vi "Phase III monitor screen.vi"() -> ()   [LabVIEW 2022 SP3]
panel:
  out "C bottom open circuit - LOX":bool
  out "C top open circuit -LOX":bool
  out "B top open circuit - LOX":bool
  out "B Top Open circuit - LOX":bool
  out "A bottom open circuit -LOX":bool
  out "A Top Open circuit -LOX":bool
  out "C Bottom  Short Circuit - ATF 2":bool
  out "C top Short Circuit - LOX":bool
  out "B Bottom short circuit - LOX":bool
  out "B top Short circuit - LOX":bool
  out "A bottom short circuit - LOX":bool
  out "A top Short Circuit - LOX":bool
  out "Speed cmd & Response mismatch- LOX":bool
  out "Motor overload - LOX":bool
  out "Over temperature - LOX":bool
  out "Over speed - LOX":bool
  out "C Phase Short circuit - LOX":bool
  out "C Phase open circuit -LOX":bool
  out "B Phase Short circuit - LOX":bool
  out "B Phase open circuit-LOX":bool
  out "A phase short circuit-LOX":bool
  out "A Phase open circuit -LOX":bool
  in  "Ia,ph,Mean  5":dbl format="%#_g A"
  in  "Ia,ph,Mean  4":dbl format="%#_g A"
  in  "DC Busbar 5":dbl format="%#_g K"
  in  "Ia,ph,Mean  2":dbl format="%#_g A"
  in  "Ic,ph,rms":dbl format="%#_g A"
  in  "Ib,ph,rms":dbl format="%#_g A"
  in  "Ia,ph,rms":dbl format="%#_g A"
  in  "Idc":dbl format="%#_g A"
  in  "Vc,ph,Mean 2":dbl format="%#_g V"
  in  "Vb,ph,Mean 2":dbl format="%#_g V"
  in  "Va,ph,Mean 2":dbl format="%#_g V"
  in  "Vc,ph,rms":dbl format="%#_g V"
  in  "Vb,ph,rms 2":dbl format="%#_g V"
  in  "Va,ph,rms 2":dbl format="%#_g V"
  in  "Vdc":dbl format="%#_g V"
  in  "DC Busbar 4":dbl format="%#_g K"
  in  "DC Busbar 3":dbl format="%#_g K"
  in  "Leg3 CJ":dbl format="%#_g K"
  in  "Leg2 CJ":dbl format="%#_g K"
  in  "Leg1 CJ":dbl format="%#_g K"
  in  "Ia,ph,Mean  3":dbl format="%#_g A"
  in  "Ia,ph,Mean  2":dbl format="%#_g A"
  in  "DC Busbar 2":dbl format="%#_g K"
  out "C bottom open circuit - ATF":bool
  out "C top open circuit -ATF":bool
  out "B top open circuit - ATF":bool
  out "B Top Open circuit - ATF":bool
  out "A bottom open circuit -ATF":bool
  out "A Top Open circuit -ATF":bool
  out "C Bottom  Short Circuit - ATF":bool
  out "C top Short Circuit - ATF":bool
  out "B Bottom short circuit - ATF":bool
  out "B top Short circuit - ATF":bool
  out "A bottom short circuit - ATF":bool
  out "A top Short Circuit - ATF":bool
  out "Speed cmd & Response mismatch- ATF":bool
  out "Motor overload - ATF":bool
  out "Over temperature - ATF":bool
  out "Over speed - ATF":bool
  out "C Phase Short circuit - ATF":bool
  out "C Phase open circuit -ATF":bool
  out "B Phase Short circuit - ATF":bool
  out "B Phase open circuit-ATF":bool
  out "A phase short circuit-ATF":bool
  out "A Phase open circuit -ATF":bool
  in  "Ia,ph,Mean":dbl format="%#_g A"
  in  "Ic,ph,rms":dbl format="%#_g A"
  in  "Ib,ph,rms":dbl format="%#_g A"
  in  "Ia,ph,rms":dbl format="%#_g A"
  in  "Idc":dbl format="%#_g A"
  in  "Vc,ph,Mean":dbl format="%#_g V"
  in  "Vb,ph,Mean":dbl format="%#_g V"
  in  "Va,ph,Mean":dbl format="%#_g V"
  in  "Vc,ph,rms":dbl format="%#_g V"
  in  "Vb,ph,rms":dbl format="%#_g V"
  in  "Va,ph,rms":dbl format="%#_g V"
  in  "Vdc":dbl format="%#_g V"
  in  "DC Busbar":dbl format="%#_g K"
  in  "DC Busbar":dbl format="%#_g K"
  in  "Leg3 CJ":dbl format="%#_g K"
  in  "Leg2 CJ":dbl format="%#_g K"
  in  "Leg1 CJ":dbl format="%#_g K"
  out "Master - Slave Failure":bool
  out "Over Power Detection":bool
  out "Over Current Detection":bool
  out "Over Voltage Detection":bool
  out "Power fail Status":bool
  out "Drive atf Health 4":bool
  out "Drive atf Health 3":bool
  out "No. of Slave Devices":dbl
  in  "Terminal Power":dbl format="%#_g W"
  in  "Terminal Current":dbl format="%#_g A"
  in  "Terminal Voltage":dbl format="%#_g V"
  in  "EXIT":bool
  # "VERSION NUMBER : 1.2"
  # "PHASE III- MONITORING GUI 1"
  # "RELEASE DATE :10/06/2024"
  # "Critical Parameters"
  # "PPSU Responses & Feedback"
  # "Thermal Data"
  # "Drive LOX Critical Parameters"
  # "Drive ATF Critical Parameters"
  # "Pressure Data"
  # "Critical Data"
  # "Drive ATF Fault Status"
  # "Drive LOX Fault Status"
  # "A-Phase top\nMOSFET Open circuit"
  # "A-Phase top MOSFET Short circuit"
  # "A-Phase top\nMOSFET Open circuit"
  # "A-Phase top MOSFET Short circuit"
  # "A-Phase open circuit"
  # "A-Phase open circuit"
  # "A-Phase Short circuit"
  # "A-Phase Short circuit"
  # "A-Phase bottom MOSFET Open circuit"
  # "A-Phase bottom MOSFET Open circuit"
  # "A-Phase bottom MOSFET Short circuit"
  # "A-Phase bottom MOSFET Short circuit"
  # "B-Phase Open circuit"
  # "B-Phase Open circuit"
  # "Vibration Data"
  # "B-Phase top MOSFET Short circuit"
  # "B-Phase top MOSFET Short circuit"
  # "B-Phase Short circuit"
  # "B-Phase Short circuit"
  # "B-Phase top MOSFET Open circuit"
  # "B-Phase top MOSFET Open circuit"
  # "C-Phase Open circuit"
  # "C-Phase Open circuit"
  # "B-Phase Bottom MOSFET Short circuit"
  # "B-Phase Bottom MOSFET Short circuit"
  # "B-Phase Bottom MOSFET Open circuit"
  # "B-Phase Bottom MOSFET Open circuit"
  # "C-Phase Short circuit"
  # "C-Phase Short circuit"
  # "C-Phase top MOSFET Open circuit"
  # "C-Phase top MOSFET Open circuit"
  # "C-Phase top MOSFET Short circuit"
  # "Over speed"
  # "C-Phase top MOSFET Short circuit"
  # "Over speed"
  # "Other Data"
  # "Over Temperature"
  # "Over Temperature"
  # "C-Phase Bottom MOSFET Open circuit"
  # "C-Phase Bottom MOSFET Short circuit"
  # "C-Phase Bottom MOSFET Open circuit"
  # "C-Phase Bottom MOSFET Short circuit"
  # "Motor Overload"
  # "Motor Overload"
  # "Speed Command & response mismatch"
  # "Speed Command & response mismatch"
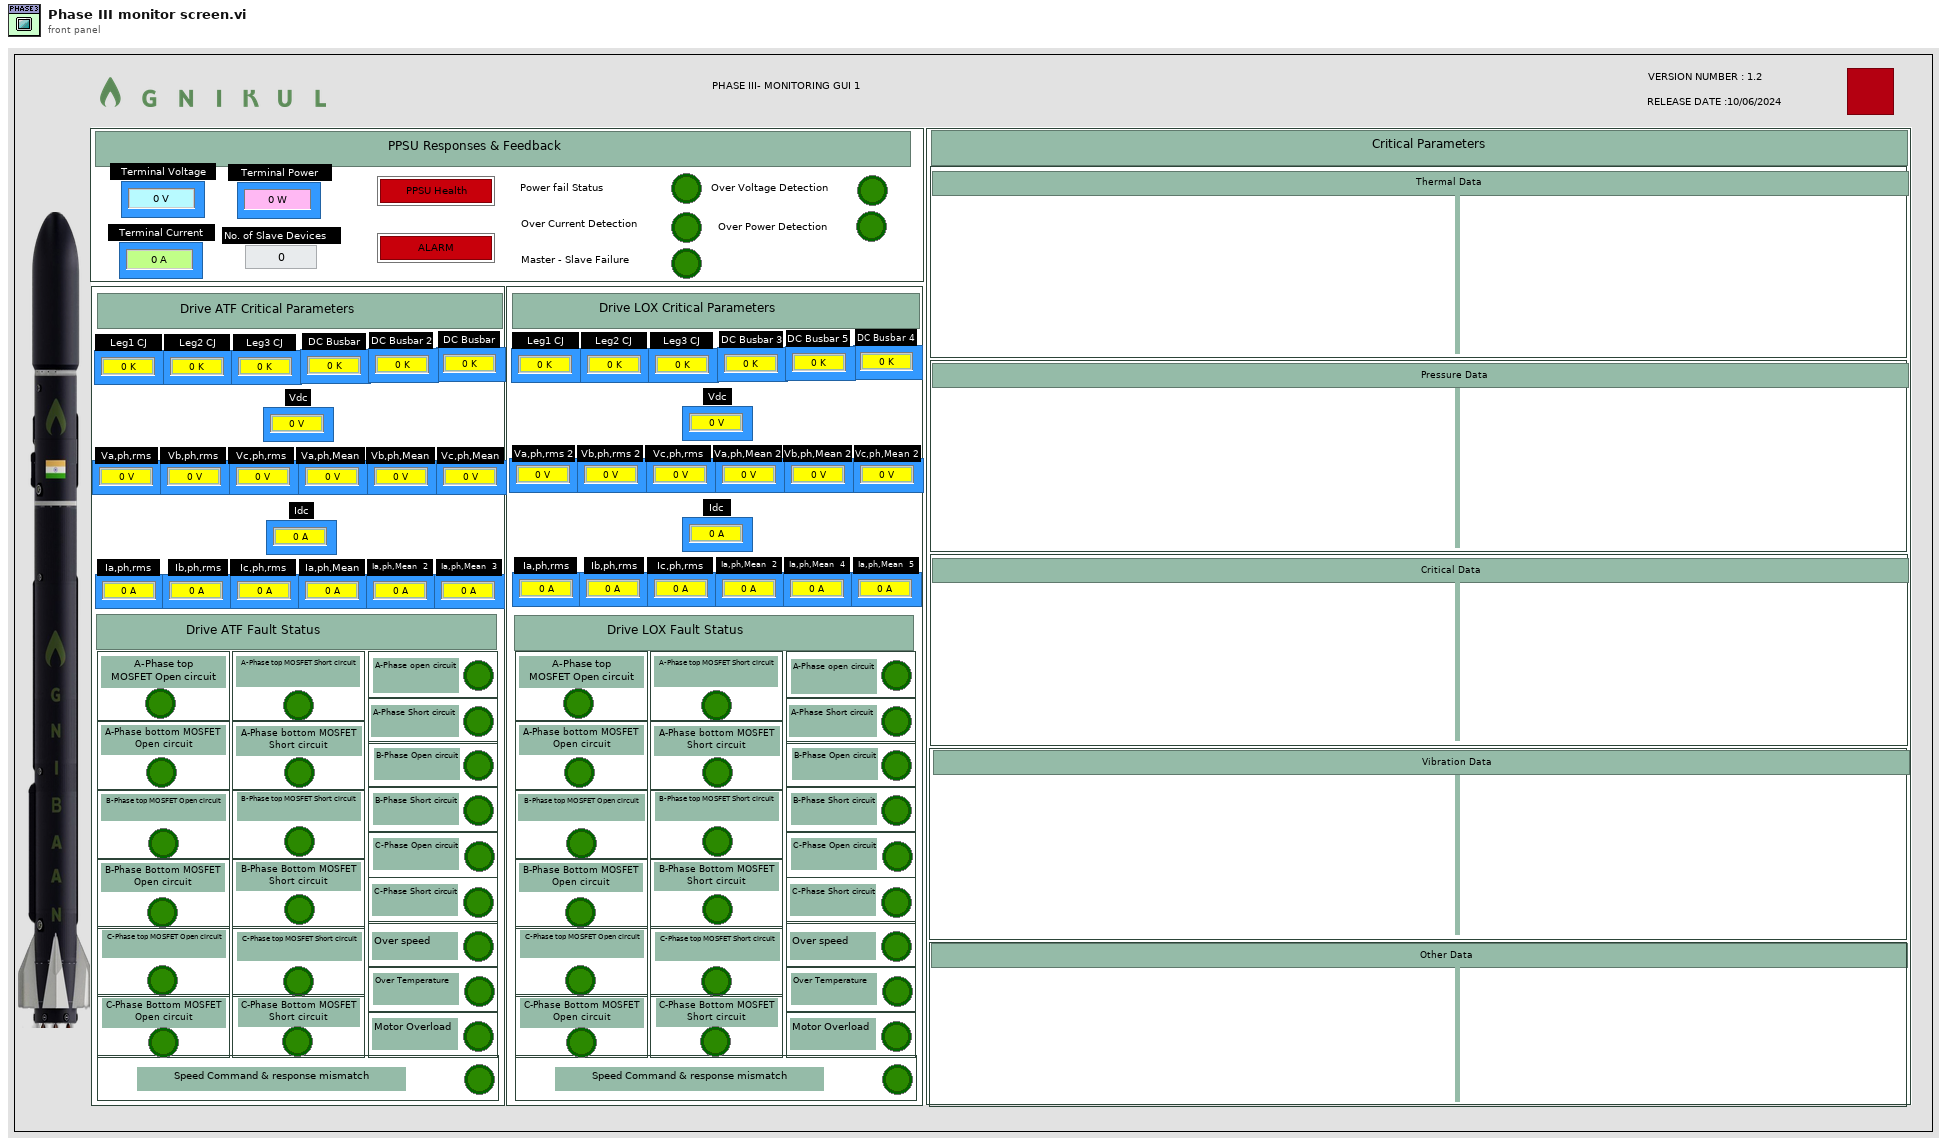
[diagram p1: front panel]
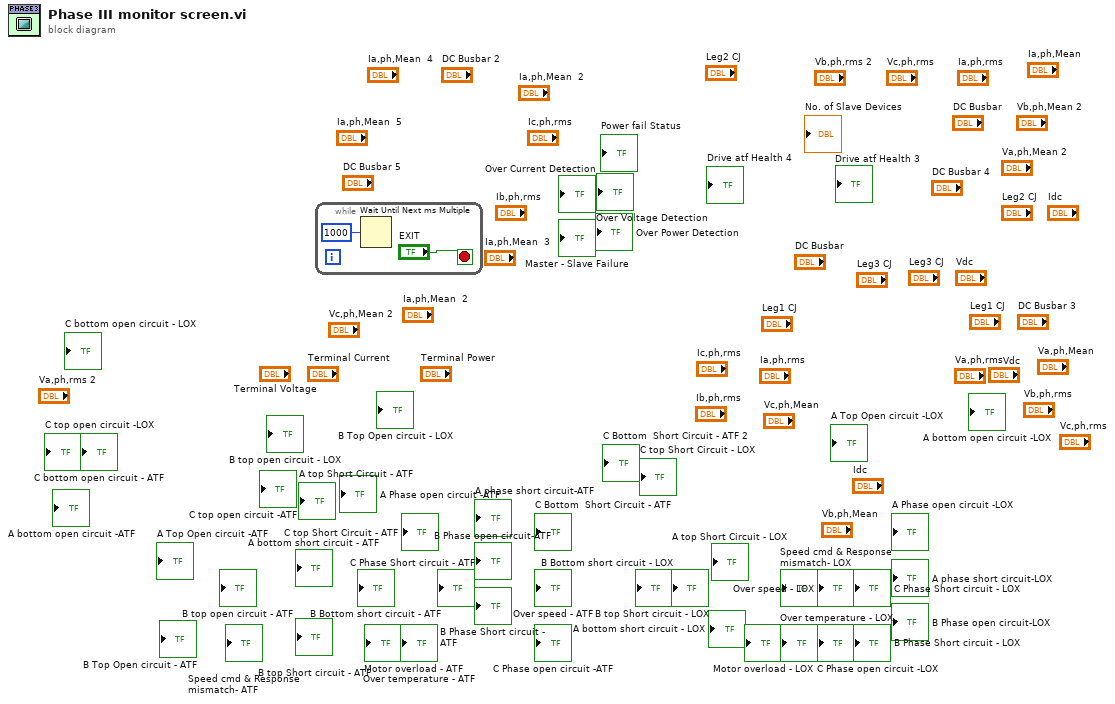
[diagram p0: block diagram]
diagram:
  n1 = while {
    stop <- "EXIT" stop-if-true
    n2 = Wait Until Next ms Multiple(millisecond multiple=u32 1000) -> ()  [unwired: 1 out]
  }
